vi "Main_Coordinate_VI.vi"(6 "Matches (real-world)":T3(array[cluster]) {"Bounding Box"."y" format="%.2f"; "Bounding Box"."x" format="%.2f"; "Score" format="%.2f"; "Scale" format="%.2f"; "Angle" format="%.2f"; "Position"."y" format="%.2f"; "Position"."x" format="%.2f"}, 7 "Mode":u16(ring) items=["Find Reference", "Update CoordSys"], 8 "error in (no error)":errorcluster, 9 "Coordinate System In":T4 {"Measurement System"."Axis Reference" items=["Direct", "Indirect"]; "Measurement System"."Angle (deg)" format="%.2f"; "Measurement System"."Origin"."Y" format="%.2f"; "Measurement System"."Origin"."X" format="%.2f"; "Reference System"."Axis Reference" items=["Direct", "Indirect"]; "Reference System"."Angle (deg)" format="%.2f"; "Reference System"."Origin"."Y" format="%.2f"; "Reference System"."Origin"."X" format="%.2f"}, 10 "Search Rect":T1={"Left"=0, "Top"=0, "Right"=2147483647, "Bottom"=2147483647, "Rotation"=0.0} {"Rotation" format="%.2f"; "Left" scale=0.0..1024.0; "Right" scale=0.0..1024.0}, 11 "Image In":T2) -> (0 "error out":errorcluster, 1 "Coordinate System Out":T4 {"Measurement System"."Axis Reference" items=["Direct", "Indirect"]; "Measurement System"."Angle (deg)" format="%.2f"; "Measurement System"."Origin"."Y" format="%.2f"; "Measurement System"."Origin"."X" format="%.2f"; "Reference System"."Axis Reference" items=["Direct", "Indirect"]; "Reference System"."Angle (deg)" format="%.2f"; "Reference System"."Origin"."Y" format="%.2f"; "Reference System"."Origin"."X" format="%.2f"}, 3 "Image Out":T2)   [LabVIEW 2015]
uses:
  <vilib>/vision/Image Controls.llb/IMAQ Image.ctl
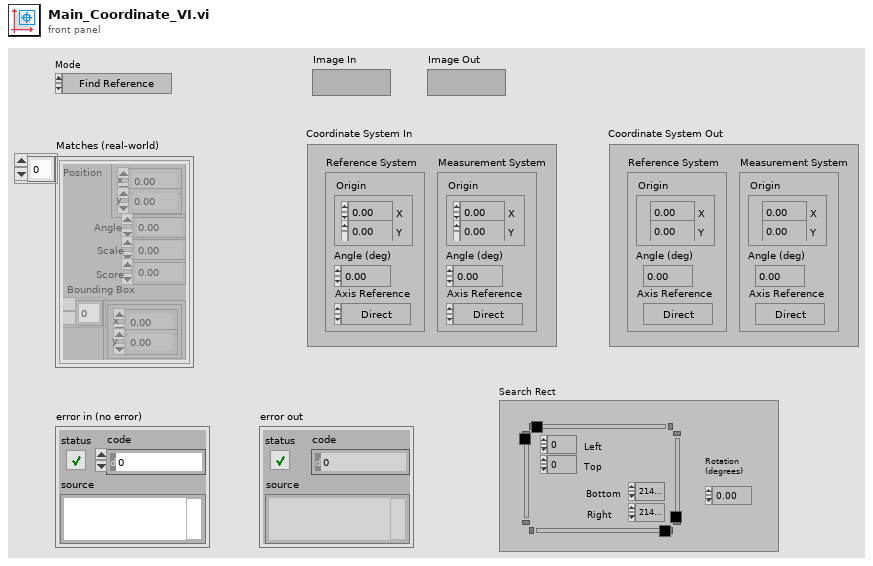
[diagram p1: front panel]
types:
  T1 = typedef "IMAQ Rectangle" = cluster{"Left":i32, "Top":i32, "Right":i32, "Bottom":i32, "Rotation":dbl}
  T2 = typedef "IMAQ Image.ctl" = refnum<image>
  T3 = cluster{"Position":cluster{"x":sgl, "y":sgl}, "Angle":sgl, "Scale":sgl, "Score":sgl, "Bounding Box":cluster{"x":sgl, "y":sgl}[]}[]
  T4 = typedef "IMAQ Coordinate System" = cluster{"Reference System":cluster{"Origin":cluster{"X":sgl, "Y":sgl}, "Angle (deg)":sgl, "Axis Reference":u32}, "Measurement System":cluster{"Origin":cluster{"X":sgl, "Y":sgl}, "Angle (deg)":sgl, "Axis Reference":u32}}
  T5 = cluster{"Show Search Area":bool, "Show Feature Found":bool, "Show Result":bool}
  T6 = cluster{"Position":cluster{"x":sgl, "y":sgl}, "Angle":sgl, "Scale":sgl, "Score":sgl, "Bounding Box":cluster{"x":sgl, "y":sgl}[]}
  T7 = cluster{"Bounding Box[0]":cluster{"x":sgl, "y":sgl}, "Bounding Box[1]":cluster{"x":sgl, "y":sgl}, "Bounding Box[2]":cluster{"x":sgl, "y":sgl}, "Bounding Box[3]":cluster{"x":sgl, "y":sgl}, "Bounding Box[4]":cluster{"x":sgl, "y":sgl}, "Bounding Box[5]":cluster{"x":sgl, "y":sgl}, "Bounding Box[6]":cluster{"x":sgl, "y":sgl}, "Bounding Box[7]":cluster{"x":sgl, "y":sgl}, "Bounding Box[8]":cluster{"x":sgl, "y":sgl}}
  T8 = cluster{"Bounding Box[3]":cluster{"x":sgl, "y":sgl}, "Bounding Box[2]":cluster{"x":sgl, "y":sgl}}
  T9 = cluster{"Bounding Box[3]":cluster{"x":sgl, "y":sgl}, "Bounding Box[0]":cluster{"x":sgl, "y":sgl}}
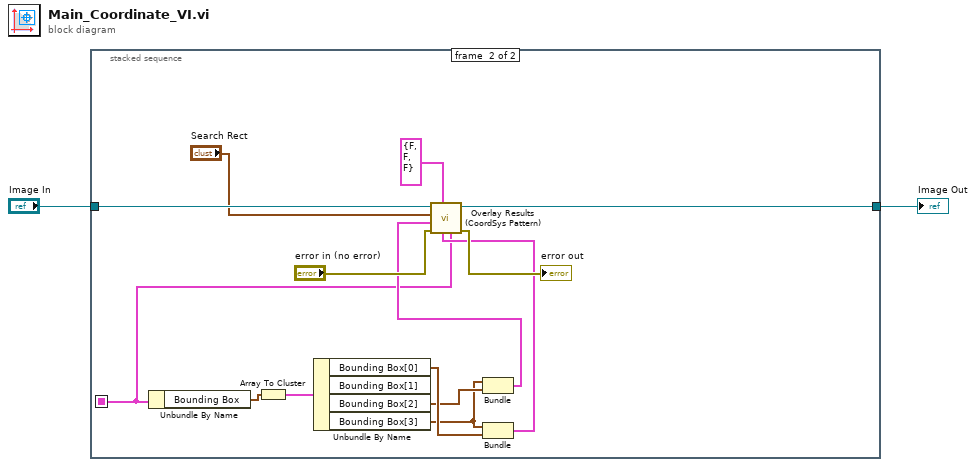
[diagram p0: block diagram]
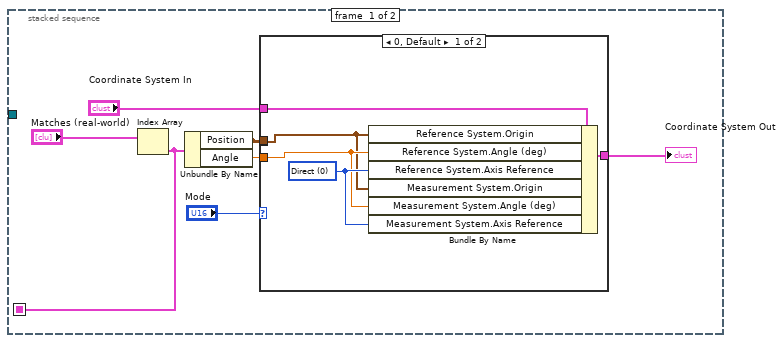
[diagram p2: hidden frame]
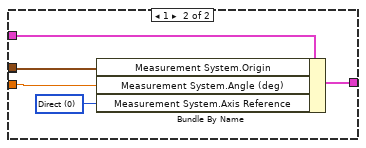
[diagram p3: hidden frame]
diagram:
  n1 = stacked-sequence {
    seq-local: [w3 _] -> [_ w22]
    tunnel: "Image In" -> [_ w33]
    tunnel: [_ w30] -> w1
    frame #0 {
      n2 = Index Array(array="Matches (real-world)") -> (element=w3:T6)  [unwired: 1 in]
      n3 = Unbundle By Name(w3) -> ("Position"=w5:cluster{"x":sgl, "y":sgl}, "Angle"=w7:sgl)
      n4 = case shown="0, Default" "Mode" {
        tunnel: w5 -> [w10 w16]
        tunnel: [w14 w19] -> w8
        tunnel: w7 -> [w11 w15]
        tunnel: "Coordinate System In" -> [w13 w18]
        tunnel: w5 -> [_ _]
        frame 0, Default {
          w12 = u32 0 items=["Direct", "Indirect"] ("Axis Reference")
          n5 = Bundle By Name(cluster=w13, "Reference System.Origin"=w10, "Reference System.Angle (deg)"=w11, "Reference System.Axis Reference"=w12, "Measurement System.Origin"=w10, "Measurement System.Angle (deg)"=w11, "Measurement System.Axis Reference"=w12) -> (w14:T4)
        }
        frame 1 {
          w17 = u32 0 items=["Direct", "Indirect"] ("Axis Reference")
          n6 = Bundle By Name(cluster=w18, "Measurement System.Origin"=w16, "Measurement System.Angle (deg)"=w15, "Measurement System.Axis Reference"=w17) -> (w19:T4)
        }
      }
      "Coordinate System Out" <- w8
    }
    frame #1 {
      n7 = Unbundle By Name(w22) -> ("Bounding Box"=w20:cluster{"x":sgl, "y":sgl}[])
      n8 = Array To Cluster(array=w20) -> (cluster=w28:T7)
      n9 = Unbundle By Name(w28) -> ("Bounding Box[0]"=w27:cluster{"x":sgl, "y":sgl}, "Bounding Box[2]"=w26:cluster{"x":sgl, "y":sgl}, "Bounding Box[3]"=w25:cluster{"x":sgl, "y":sgl})  [unwired: 1 out]
      n10 = Bundle("Bounding Box[3]"=w25, "Bounding Box[2]"=w26) -> (w24:T8)  [unwired: 1 in]
      n11 = Bundle("Bounding Box[3]"=w25, "Bounding Box[0]"=w27) -> (w23:T9)  [unwired: 1 in]
      n12 = call <vilib>:"Overlay Results (CoordSys Pattern).vi"("Match"=w22, "Axis 2"=w23, "Setup"=T5 {"Show Search Area"=FALSE, "Show Feature Found"=FALSE, "Show Result"=FALSE}, "error in (no error)"="error in (no error)", "Axis 1"=w24, "Search Rect"="Search Rect", "Image In"=w33) -> ("error out"=→"error out":errorcluster, "Image Out"=w30:T2)  [unwired: 3 out]
    }
  }
  "Image Out" <- w1
